vi "PMTreadwrite.vi"(7 "Enum":enum16{"READ", "WRITE"}(ring)=enum."WRITE", 8 "error in":errorcluster, 11 "PMT Settings":cluster{"Bin Length":dbl, "Show Mean":bool}={"Bin Length"=100.0, "Show Mean"=FALSE}) -> (0 "error out":errorcluster, 3 "Count Chart":u32(graph))   [LabVIEW 2019]
uses:
  <vilib>/Analysis/baseanly.llb/Mean (DBL).vi
  <vilib>/Utility/error.llb/Error Cluster From Error Code.vi
  <vilib>/rvi/errors/niLvFpgaAdjustHostInterfaceError.vi
  <vilib>/rvi/interface/nirviReadWriteControl/nirviReadWriteControl.xnode
  <vilib>/rvi/interface/Simulation/niFpgaSimulationCallBeginRW.vi
  <vilib>/Analysis/NI_AALBase.lvlib
  NiFpgaLv.dll
panel:
  out "PMT saturation 2":bool
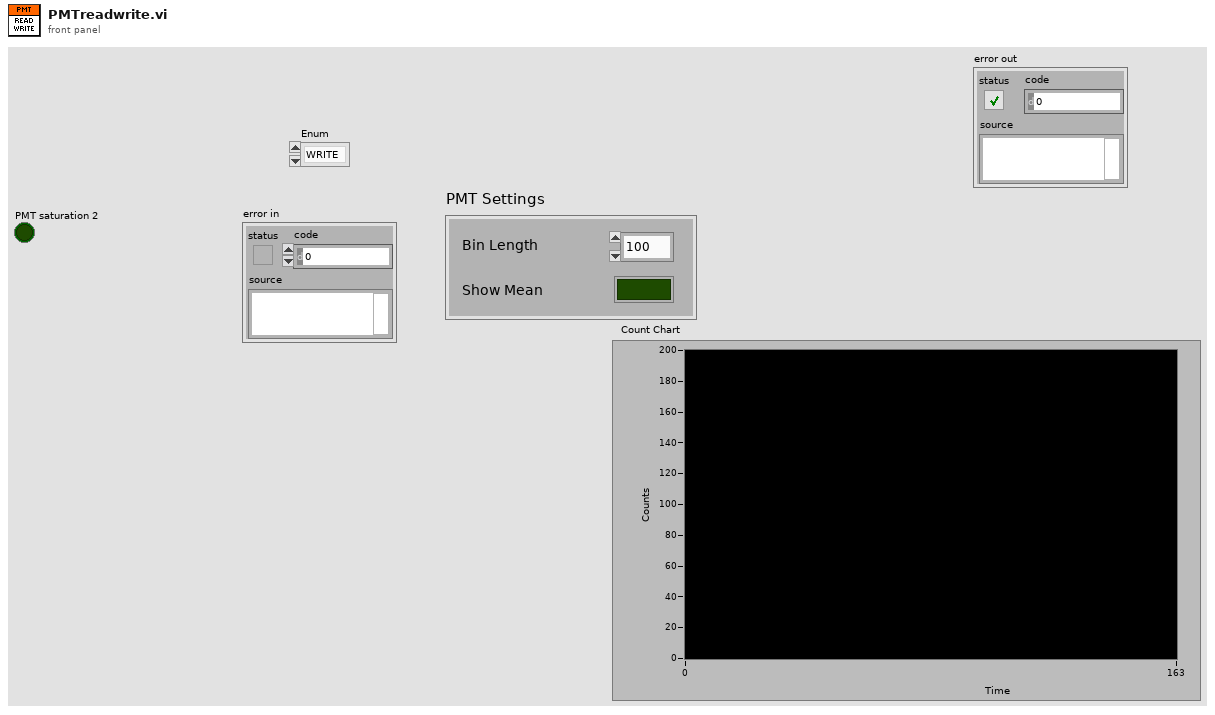
[diagram p1: front panel]
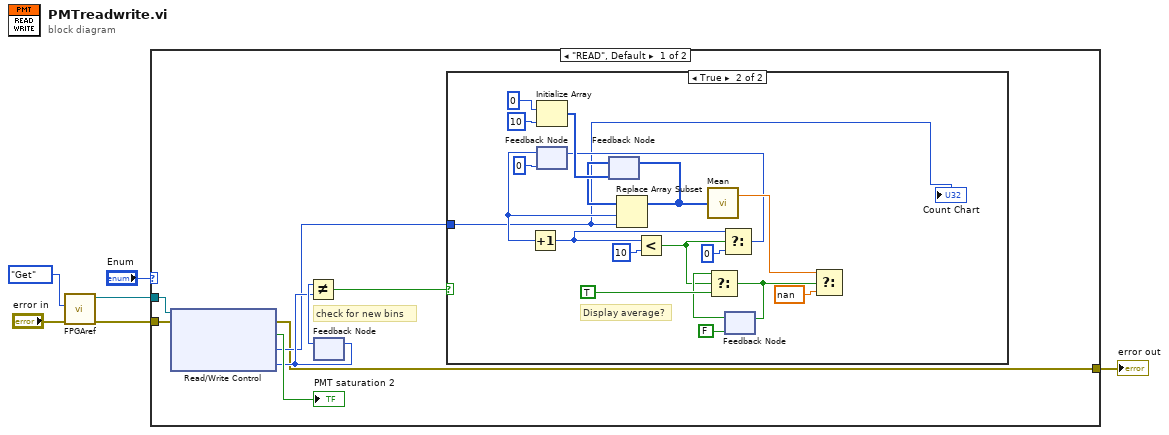
[diagram p0: block diagram]
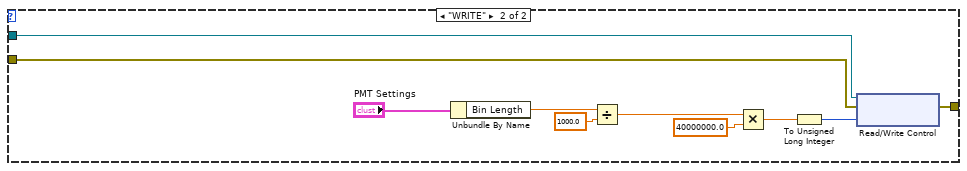
[diagram p3: hidden frame]
diagram:
  n1 = call "FPGAref.vi"("error in"="error in", "Enum"=enum16{"Set", "Get"}."Get") -> ("error out"=w3:errorcluster, "FPGA VI Reference Out 2"=w4:refnum<k20>)  [unwired: 4 in]
  n2 = case shown="\"READ\", Default" "Enum" {
    tunnel: w4 -> [w9 w42]
    tunnel: w3 -> [w8 w41]
    tunnel: [w7 w34] -> w1
    frame "READ", Default {
      # "check for new bins"
      n3 = xnode "Read/Write Control"("FPGA VI Reference In"=w9, "error in"=w8) -> ("error out"=w7:errorcluster, "PMT saturation"=→"PMT saturation 2":bool, "Frequency Chart"=w10:u32, "bin number"=w12:u32)  [unwired: 1 out]
      n4 = feedback #1() -> (w13:u32)  [unwired: 1 in]
      n5 = Not Equal?(x=w13, y=w12) -> (x != y?=w11:bool)
      n6 = feedback-in #1(w12) -> ()
      n7 = case shown="True" w11 {
        tunnel: w10 -> [_ w15]
        frame False {
        }
        frame True {
          # "Display average?"
          n8 = Initialize Array(u32 0 ("Frequency Chart"), 10 ("dimension size")) -> (w31:u32[])
          n9 = feedback #2(0) -> (w25:i32)
          n10 = Increment(x=w25) -> (x+1=w22:i32)
          n11 = feedback #3(w31) -> (w30:u32[])
          n12 = Replace Array Subset(array=w30, new element=w15, index=w25) -> (w29:u32[])
          n13 = feedback-in #3(w29) -> ()
          n14 = Less?(x=w22, y=10) -> (x < y?=w17:bool)
          n15 = call-poly <vilib>:"Mean.vi"("X"=w29) -> ("mean"=w28:dbl)  [unwired: 1 out]
          n16 = Select(t=w22, s=w17, f=0) -> (s? t:f=w21:i32)
          n17 = feedback-in #2(w21) -> ()
          n18 = feedback #4(FALSE) -> (w18:bool)
          n19 = Select(t=w18, s=w17, f=TRUE) -> (s? t:f=w16:bool)
          n20 = feedback-in #4(w16) -> ()
          n21 = Select(t=w28, s=w16, f=nan) -> ()  [unwired: 1 out]
          "Count Chart" <- w15
        }
      }
    }
    frame "WRITE" {
      n22 = Unbundle By Name("PMT Settings") -> ("Bin Length"=w37:dbl)
      n23 = Divide(x=w37, y=1000.0) -> (x/y=w39:dbl)
      n24 = Multiply(x=w39, y=40000000.0) -> (x*y=w36:dbl)
      n25 = To Unsigned Long Integer(number=w36) -> (unsigned 32bit integer=w35:u32)
      n26 = xnode "Read/Write Control"("FPGA VI Reference In"=w42, "error in"=w41, "ticks per bin"=w35) -> ("error out"=w34:errorcluster)  [unwired: 1 out]
    }
  }
  "error out" <- w1
